vi "Build Method List.vi"(8 "error in (no error)":errorcluster, 9 "Method List (VEnum)":variant) -> (0 "error out":errorcluster, 3 "PyObjects":T1[](array[typedef]))   [LabVIEW 2020, in "jki_python_bridge.lvlib" / "Server.lvclass"]
uses:
  Server.lvclass
  Type Definitions/Python Object and Method Names - Cluster.ctl
  Type Definitions/Python Method.ctl
  <userlib>/_OpenG.lib/array/array.llb/Conditional Auto-Indexing Tunnel (String)__ogtk.vi
  <userlib>/_OpenG.lib/array/array.llb/Remove Duplicates from 1D Array (String)__ogtk.vi
  <userlib>/_OpenG.lib/array/array.llb/Search 1D Array (String)__ogtk.vi
  <userlib>/_OpenG.lib/array/array.llb/Index 1D Array Elements (String)__ogtk.vi
  <userlib>/_OpenG.lib/lvdata/lvdata.llb/openg_variant.lvlib
  <userlib>/_OpenG.lib/error/error.llb/openg_error.lvlib
  <userlib>/_OpenG.lib/array/array.llb/openg_array.lvlib
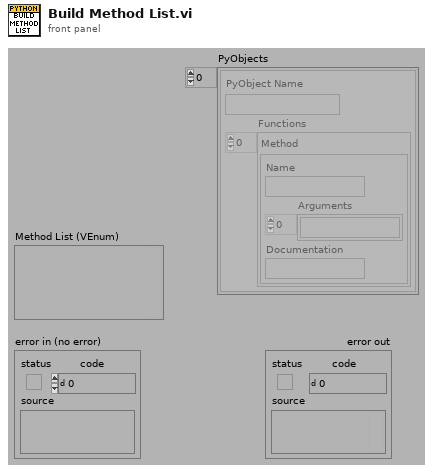
[diagram p1: front panel]
types:
  T1 = typedef "jki_python_bridge.lvlib/Server.lvclass/Python Object and Method Names - Cluster.ctl" = cluster{"PyObject Name":string, "Functions":T2[]}
  T2 = typedef "jki_python_bridge.lvlib/Server.lvclass/Python Method.ctl" = cluster{"Name":string, "Arguments":string[], "Documentation":string}
  T3 = typedef "openg_variant.lvlib/Type Descriptor Enumeration__ogtk.ctl" = enum8{"<Null>", "I8", "I16", "I32", "I64", "U8", "U16", "U32", "U64", "SGL", "DBL", "EXT", "CSG", "CDB", "CXT", "0x0F", "0x10", "0x11", "0x12", "0x13", "0x14", "Enum U8", "Enum U16", "Enum U32", "Enum U64", "SGL PQ", "DBL PQ", "EXT PQ", "CSG PQ", "CDB PQ", "CXT PQ", "0x1F", "0x20", "Boolean", "0x22", "0x23", "0x24", "0x25", "0x26", "0x27", "0x28", "0x29", "0x2A", "0x2B", "0x2C", "0x2D", "0x2E", "0x2F", "String", "0x31", "Path", "Pict", "0x34", "0x35", "0x36", "DAQ", "0x38", "0x39", "0x3A", "0x3B", "0x3C", "0x3D", "0x3E", "0x3F", "Array", "0x41", "0x42", "0x43", "0x44", "0x45", "0x46", "0x47", "0x48", "0x49", "0x4A", "0x4B", "0x4C", "0x4D", "0x4E", "0x4F", "Cluster", "0x51", "0x52", "Variant", "Waveform", "0x55", "0x56", "0x57", "0x58", "0x59", "0x5A", "0x5B", "0x5C", "0x5D", "0x5E", "Fixed Point", "0x60", "0x61", "0x62", "0x63", "0x64", "0x65", "0x66", "0x67", "0x68", "0x69", "0x6A", "0x6B", "0x6C", "0x6D", "0x6E", "0x6F", "Refnum", "0x71", "0x72", "Set Collection", "Map Collection"}
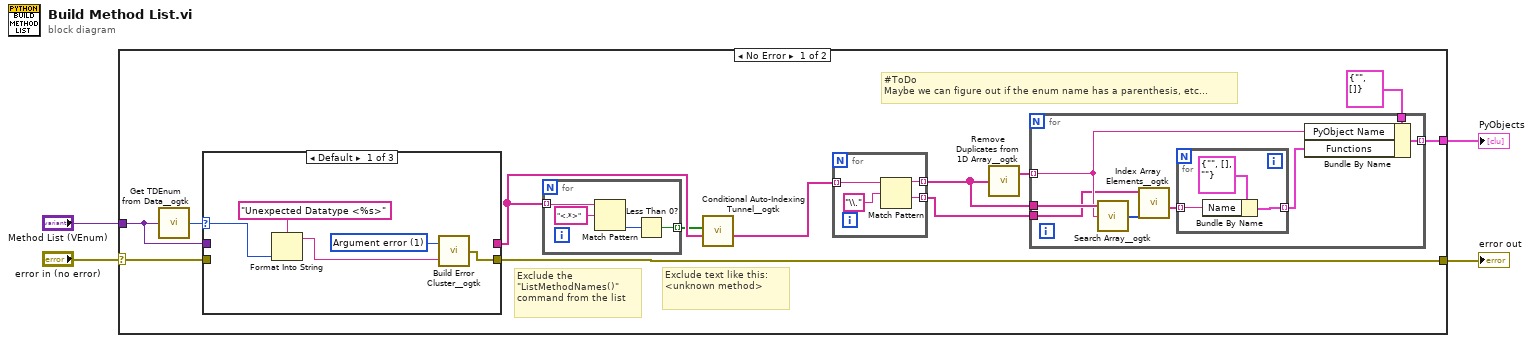
[diagram p0: block diagram]
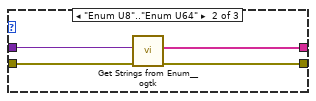
[diagram p2: hidden frame]
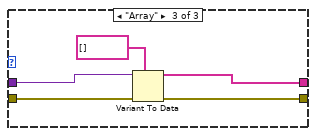
[diagram p3: hidden frame]
diagram:
  n1 = case shown="No Error" "error in (no error)" {
    selector: "error in (no error)" -> [w14 w50]
    tunnel: [w11 w50] -> w3
    tunnel: [w8 _] -> w2
    tunnel: "Method List (VEnum)" -> [w16 _]
    frame No Error {
      # "#ToDo\nMaybe we can figure out if the enum name has a parenthesis, etc..."
      # "Exclude text like this: <unknown method>"
      # "Exclude the \"ListMethodNames()\" command from the list"
      n2 = call <userlib>:"Get TDEnum from Data__ogtk.vi"("Data"=w16) -> ("Type Descriptor Enumeration"=w15:T3)  [unwired: 4 in]
      n3 = case shown="Default" w15 {
        selector: w15 -> [w36 _ _]
        tunnel: [_ w44 w49] -> w13
        tunnel: [w37 w43 w48] -> w11
        tunnel: w14 -> [_ w42 w47]
        tunnel: w16 -> [_ w41 w46]
        frame Default {
          w40 = 1 items=["No error", "Argument error", "Memory is full", "Out of zone", "End of file", "File already open", "Generic file I/O error", "File not found", "File permission error", "Disk is full", "Duplicate path", "Too many files open", "System feature not enabled", "Resource file not found", "Cannot add resource", "Resource not found", "Image not found", "Image memory error", "Pen does not exist", "Config type invalid", "Config token not found", "Config parse error", "Config memory error", "Bad external code format", "Bad external code offset", "External code not present", "Null window", "Destroy window error", "Null menu", "Print aborted", "Bad print record", "Print driver error", "Windows error during printing", "Memory error during printing", "Print dialog error", "Generic print error", "Invalid device refnum", "Device not found", "Device parameter error", "Device unit error", "Cannot open device", "Device call aborted", "Generic error", "Cancelled by user", "Object ID too low", "Object ID too high", "Object not in heap", "Unknown heap", "Unknown object (invalid DefProc)", "Unknown object (DefProc not in table)", "Message out of range", "Invalid (null) method", "Unknown message", "Manager call not supported", "Bad address", "Network operation in progress", "Network operation timed out", "Connection is busy", "Network attribute not supported", "Network error", "Address in use", "System out of memory", "Connection aborted", "Connection refused", "Not connected", "Already connected", "Connection closed", "Initialization error (interapplication manager)", "Bad occurrence", "Wait on unbound occurrence handler", "Occurrence queue overflow", "Datalog type conflict", "Unused", "Unrecognized type (interapplication manager)", "Memory corrupt", "Failed to make temporary DLL", "Old CIN version", "Drag socket not found", "Failed to load drop-object", "Failed to register OLE object", "Failed to release OLE object", "Format specifier type mismatch", "Unknown format specifier", "Too few format specifiers", "Too many format specifiers", "Scan failed", "Newer CIN version", "Error converting to variant", "Runtime menu error", "Password tampered", "Variant attribute not found", "Incompatible variant data type", "Event data is not available", "Event Store is not present", "Occurrence is not found", "Event Queue is not created", "Event info is not available", "Refnum passed is NULL", "Error retrieving Class GUID", "Error retrieving CoClass GUID", "Error retrieving TypeLib GUID.", "Bad built application magic bytes.", "Specific driver is different from the specific driver associated with the Logical Name.", "There is no session opened to the class driver.", "Max Error", "MAX - Error with config objects", "MAX - Error loading configuration", "MAX - Group not supported"]
          n4 = Format Into String(format string="Unexpected Datatype <%s>" ("Format String"), w36) -> (resulting string=w38:string)  [unwired: 2 in, 1 out]
          n5 = call <userlib>:"Build Error Cluster__ogtk.vi"("String to Prepend to source (\"\")"=w38, "code"=w40) -> ("error out"=w37:errorcluster)
        }
        frame "Enum U8".."Enum U64" {
          n6 = call <userlib>:"Get Strings from Enum__ogtk.vi"("error in (no error)"=w42, "Enum"=w41) -> ("error out"=w43:errorcluster, "Enum Strings"=w44:string[])  [unwired: 6 in, 2 out]
        }
        frame "Array" {
          n7 = Variant To Data(error in=w47, type=string[] [] ("Functions"), Variant=w46) -> (data=w49:string[], error out=w48:errorcluster)
        }
      }
      n8 = for {
        tunnel: w13 -> [w35] mode=indexing
        tunnel: [w32] -> w12 mode=indexing
        n9 = Match Pattern(string=w35, regular expression="<.*>") -> (offset past match=w33:i32)  [unwired: 1 in, 3 out]
        n10 = Less Than 0?(x=w33) -> (x < 0?=w32:bool)
      }
      n11 = call-poly <userlib>:"Conditional Auto-Indexing Tunnel__ogtk.vi"("Array in"=w13, "Elements to keep"=w12) -> ("Filtered Array out"=w10:string[])  [unwired: 5 in]
      n12 = for {
        tunnel: w10 -> [w30] mode=indexing
        tunnel: [w29] -> w6 mode=indexing
        tunnel: [w28] -> w5 mode=indexing
        n13 = Match Pattern(string=w30, regular expression="\\.") -> (before substring=w29:string, after substring=w28:string)  [unwired: 1 in, 2 out]
      }
      n14 = call-poly <userlib>:"Remove Duplicates from 1D Array__ogtk.vi"("Input Array"=w6) -> ("Output Array"=w9:string[])  [unwired: 1 out]
      n15 = for {
        tunnel: w9 -> [w22] mode=indexing
        tunnel: w6 -> [w23]
        tunnel: [w21] -> w8 mode=indexing
        tunnel: T1 {"PyObject Name"="", "Functions"=[]} ("PyObject") -> [w20]
        tunnel: w5 -> [w19]
        n16 = call-poly <userlib>:"Search Array__ogtk.vi"("Array"=w23, "Element Data"=w22) -> ("Indices of Elements"=w24:i32[])  [unwired: 7 in]
        n17 = call-poly <userlib>:"Index Array Elements__ogtk.vi"("indices"=w24, "array"=w19) -> ("elements"=w18:string[])  [unwired: 9 in]
        n18 = for {
          tunnel: w18 -> [w27] mode=indexing
          tunnel: [w26] -> w17 mode=indexing
          n19 = Bundle By Name(cluster=T2 {"Name"="", "Arguments"=[], "Documentation"=""} ("Functions 2"), "Name"=w27) -> (w26:T2)
        }
        n20 = Bundle By Name(cluster=w20, "PyObject Name"=w22, "Functions"=w17) -> (w21:T1)
      }
    }
    frame Error {
    }
  }
  "error out" <- w3
  "PyObjects" <- w2
